vi "DataString.vi"(1 "Value":string, 2 "Item":string="Data") -> (0 "String":string)   [LabVIEW 2014]
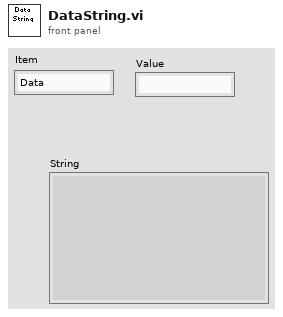
[diagram p1: front panel]
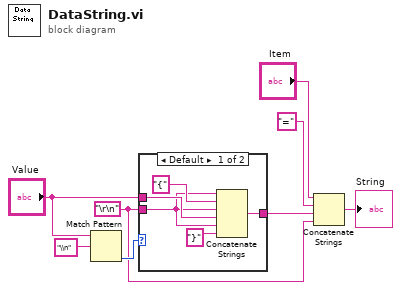
[diagram p0: block diagram]
diagram:
  w1 = "\r\n"
  n1 = Match Pattern(string="Value", regular expression="\\n") -> (offset past match=w5:i32)  [unwired: 1 in, 3 out]
  n2 = case shown="Default" w5 {
    tunnel: "Value" -> [w12 w14]
    tunnel: [w9 w14] -> w3
    tunnel: w1 -> [w11 _]
    frame Default {
      n3 = Concatenate Strings(w11, "{" ("string"), w11, w12, w11, "}" ("string")) -> (w9:string)
    }
    frame -1 {
    }
  }
  n4 = Concatenate Strings("Item", "=" ("string"), w3, w1) -> (→"String":string)
